vi "Ex3_Serial_Write_Read.vi"(0 "VISA resource":refnum<visa-resource-name>="COM4", 5 "Comando":T2(ring), 7 "stop":bool, 9 "Decisión":bool, 11 "error in (no error)":errorcluster) -> (1 "Buffer Completo":string, 3 "Buffer Filtrado":string, 4 "VISA resource name out":refnum<visa-resource-name>, 6 "Señales Digitales":dynamicdata(graph), 10 "Señales Analógicas":dynamicdata(graph), 12 "LISTO?":bool=TRUE, 14 "Cluster Señales":T1, 15 "error out":errorcluster)   [LabVIEW 2020]
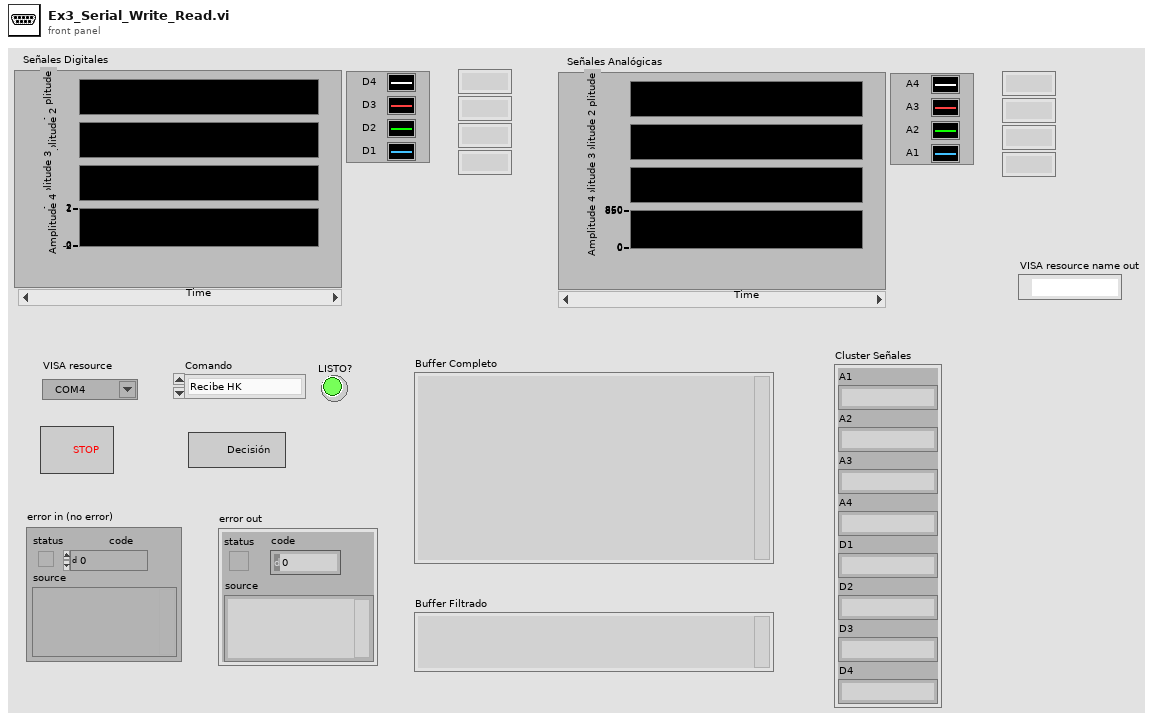
[diagram p1: front panel]
types:
  T1 = cluster{"A1":string, "A2":string, "A3":string, "A4":string, "D1":string, "D2":string, "D3":string, "D4":string}
  T2 = enum16{"Recibe HK", "Act Fecha", "Parametros", "Reset", "Stop"}
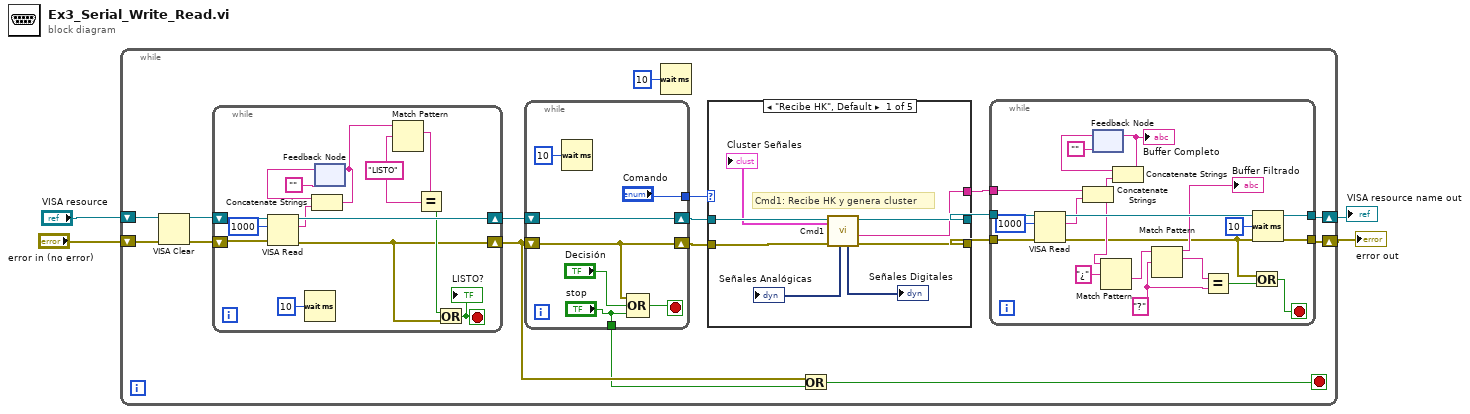
[diagram p0: block diagram]
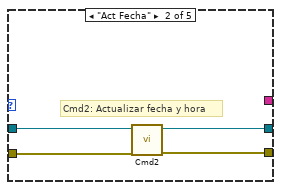
[diagram p2: hidden frame]
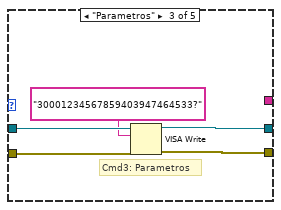
[diagram p3: hidden frame]
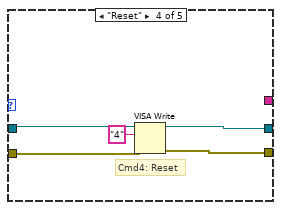
[diagram p4: hidden frame]
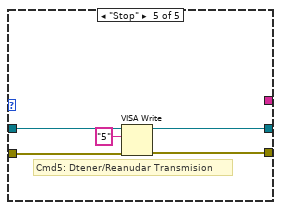
[diagram p5: hidden frame]
diagram:
  n1 = while {
    shift-right: [w8] -> w3
    shift-left: "error in (no error)" -> [w14]
    shift-right: [w9] -> w4
    shift-left: "VISA resource" -> [w16]
    stop <- w17 stop-if-true
    n2 = VISA Clear(VISA resource name=w16, error in (no error)=w14) -> (VISA resource name out=w15:refnum<visa-resource-name>, error out=w13:errorcluster)
    n3 = while {
      shift-right: [w76] -> w7
      shift-left: w13 -> [w87]
      shift-right: [w85] -> w19
      shift-left: w15 -> [w88]
      stop <- w75 stop-if-true
      w78 = "LISTO" ("regular expression")
      n4 = VISA Read(VISA resource name=w88, byte count=u32 1000, error in (no error)=w87) -> (VISA resource name out=w85:refnum<visa-resource-name>, read buffer=w84:string, error out=w76:errorcluster)  [unwired: 1 out]
      n5 = Wait (ms)(milliseconds to wait=u32 10) -> ()  [unwired: 1 out]
      n6 = feedback #1("") -> (w83:string)
      n7 = Concatenate Strings(w83, w84) -> (w80:string)
      n8 = feedback-in #1(w80) -> ()
      n9 = Match Pattern(string=w80, regular expression=w78) -> (match substring=w79:string)  [unwired: 1 in, 3 out]
      n10 = Equal?(x=w79, y=w78) -> (x = y?=w77:bool)
      n11 = Or(x=w77, y=w76) -> (x .or. y?=w75:bool)
      "LISTO?" <- w75
    }
    n12 = while {
      tunnel: ["Comando"] -> w21
      shift-right: [w46] -> w20
      shift-left: w19 -> [w46]
      shift-right: [w43] -> w18
      shift-left: w7 -> [w43]
      tunnel: ["stop"] -> w6
      stop <- w44 stop-if-true
      n13 = Wait (ms)(milliseconds to wait=u32 10) -> ()  [unwired: 1 out]
      n14 = Compound Arithmetic op=OR(w43, "Decisión", "stop") -> (w44:bool)
    }
    n15 = Wait (ms)(milliseconds to wait=u32 10) -> ()  [unwired: 1 out]
    n16 = case shown="\"Recibe HK\", Default" w21 {
      tunnel: w20 -> [w55 w59 w62 w69 w74]
      tunnel: w18 -> [w54 w58 w61 w68 w72]
      tunnel: [w52 w57 w64 w66 w73] -> w11
      tunnel: [w53 w56 w63 w67 w71] -> w10
      tunnel: [w51 _ _ _ _] -> w5
      frame "Recibe HK", Default {
        # "Cmd1: Recibe HK y genera cluster"
        n17 = call "Cmd1.vi"("error in (no error)"=w54, "VISA Refnum in"=w55) -> ("error out (no error)"=w53:errorcluster, "read buffer"=w51:string, "VISA Refnum in 2"=w52:refnum<visa-resource-name>, "Señales Digitales"=→"Señales Digitales":dynamicdata, "Señales Analógicas"=→"Señales Analógicas":dynamicdata, "Señales"=→"Cluster Señales":T1)  [unwired: 4 in]
      }
      frame "Act Fecha" {
        # "Cmd2: Actualizar fecha y hora"
        n18 = call "Cmd2.vi"("error in (no error)"=w58, "VISA Refnum in"=w59) -> ("error out"=w56:errorcluster, "VISA Refnum out"=w57:refnum<visa-resource-name>)  [unwired: 7 in, 1 out]
      }
      frame "Parametros" {
        # "Cmd3: Parametros"
        n19 = VISA Write(VISA resource name=w62, write buffer="30001234567859403947464533?", error in (no error)=w61) -> (VISA resource name out=w64:refnum<visa-resource-name>, error out=w63:errorcluster)  [unwired: 1 out]
      }
      frame "Reset" {
        # "Cmd4: Reset"
        n20 = VISA Write(VISA resource name=w69, write buffer="4", error in (no error)=w68) -> (VISA resource name out=w66:refnum<visa-resource-name>, error out=w67:errorcluster)  [unwired: 1 out]
      }
      frame "Stop" {
        # "Cmd5: Dtener/Reanudar Transmision"
        n21 = VISA Write(VISA resource name=w74, write buffer="5", error in (no error)=w72) -> (VISA resource name out=w73:refnum<visa-resource-name>, error out=w71:errorcluster)  [unwired: 1 out]
      }
    }
    n22 = Or(x=w7, y=w6) -> (x .or. y?=w17:bool)
    n23 = while {
      tunnel: w11 -> [w38]
      tunnel: w10 -> [w37]
      tunnel: [w33] -> w9
      tunnel: [w23] -> w8
      tunnel: w5 -> [w25]
      stop <- w22 stop-if-true
      w34 = "?" ("regular expression")
      n24 = VISA Read(VISA resource name=w38, byte count=u32 1000, error in (no error)=w37) -> (VISA resource name out=w33:refnum<visa-resource-name>, read buffer=w30:string, error out=w23:errorcluster)  [unwired: 1 out]
      n25 = Concatenate Strings(w25, w30) -> (w29:string)
      n26 = feedback #2("") -> (w27:string)
      n27 = Match Pattern(string=w29, regular expression="¿") -> (after substring=w39:string)  [unwired: 1 in, 3 out]
      n28 = Concatenate Strings(w27, w29) -> (w28:string)
      "Buffer Completo" <- w28
      n29 = feedback-in #2(w28) -> ()
      n30 = Match Pattern(string=w39, regular expression=w34) -> (before substring=→"Buffer Filtrado":string, match substring=w32:string)  [unwired: 1 in, 2 out]
      n31 = Equal?(x=w32, y=w34) -> (x = y?=w24:bool)
      n32 = Or(x=w23, y=w24) -> (x .or. y?=w22:bool)
      n33 = Wait (ms)(milliseconds to wait=u32 10) -> ()  [unwired: 1 out]
    }
  }
  "error out" <- w3
  "VISA resource name out" <- w4
